vi "Get UnitDB.vi"(8 "error in (no error)":errorcluster, 10 "PartNumberData":T1(array[cluster]), 11 "PreUUT in":refnum<class "PreUUT.lvclass">) -> (0 "error out":errorcluster, 3 "PreUUT out":refnum<class "PreUUT.lvclass">)   [LabVIEW 2021, in "PreUUT.lvclass"]
uses:
  PreUUT.lvclass
  PreUUT.lvclass/PreUUT.ctl
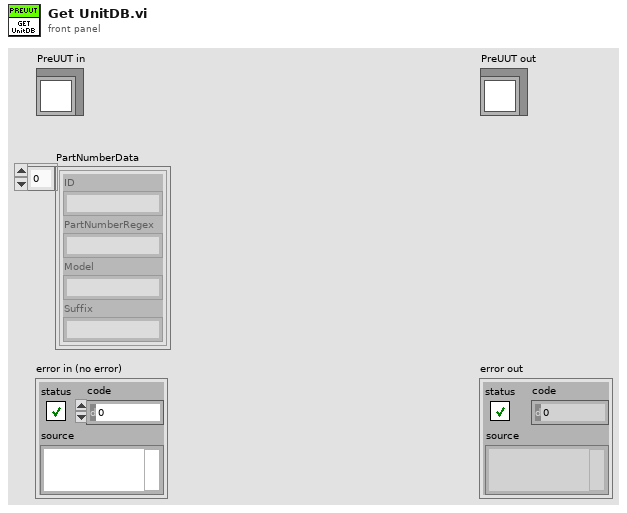
[diagram p1: front panel]
types:
  T1 = cluster{"ID":string, "PartNumberRegex":string, "Model":string, "Suffix":string}[]
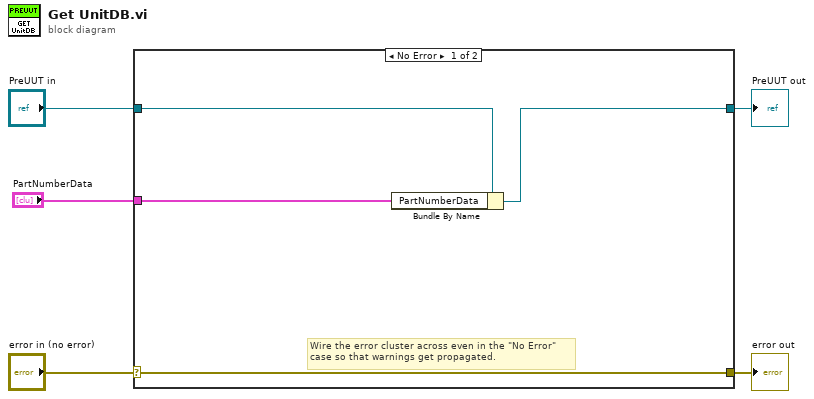
[diagram p0: block diagram]
diagram:
  n1 = case shown="No Error" "error in (no error)" {
    selector: "error in (no error)" -> [w9 w11]
    tunnel: [w9 w11] -> w4
    tunnel: [w7 w10] -> w2
    tunnel: "PreUUT in" -> [w8 w10]
    tunnel: "PartNumberData" -> [w6 _]
    frame No Error {
      # "Wire the error cluster across even in the \"No Error\"\ncase so that warnings get propagated."
      n2 = Bundle By Name(cluster=w8, "PartNumberData"=w6) -> (w7:refnum<class "PreUUT.lvclass">)
    }
    frame Error {
    }
  }
  "error out" <- w4
  "PreUUT out" <- w2
